vi "3.vi"() -> ()   [LabVIEW 2015]
panel:
  out "New":T1
  in  "Roll Number":i32
  in  "New Name":string
  in  "Old Cluster":T1
  # "Replace Name and Roll Number of Old Cluster by the New name\nand Roll Number and write to the New Cluster. The VI has a broken\nwire and you need to correct this."
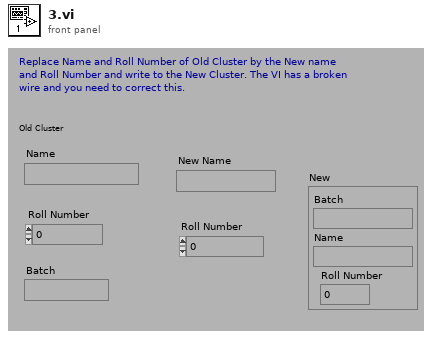
[diagram p1: front panel]
types:
  T1 = cluster{"Batch":string, "Name":string, "Roll Number":i32}
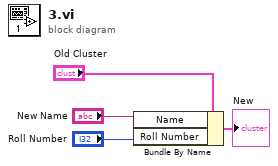
[diagram p0: block diagram]
diagram:
  n1 = Bundle By Name(cluster="Old Cluster", "Name"="New Name", "Roll Number"="Roll Number") -> (→"New":T1)
